vi "InitializeFunnelsByIndex.vi"(8 "error in (no error)":errorcluster, 10 "Funnels":string[](array[string]), 11 "Setting Database in":refnum<class "Setting Database.lvclass">) -> (0 "error out":errorcluster, 3 "Setting Database out":refnum<class "Setting Database.lvclass">)   [LabVIEW 2019, in "Setting Database.lvclass"]
uses:
  Setting Database.lvclass
  Funnel Settings/Funnel Settings.lvclass
  C:/Users/Albro/Documents/GitHub/AFM-Lithography/lvsrc/Classes/Settings/ObjectSettings/ObjectSettings.lvclass
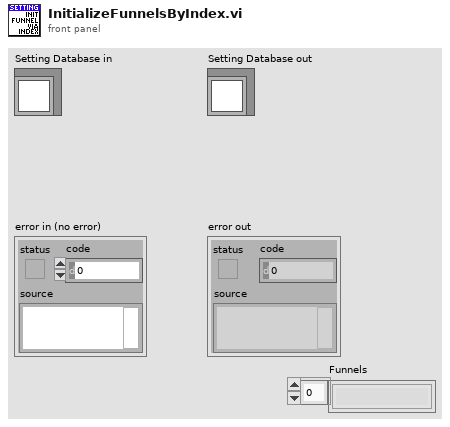
[diagram p1: front panel]
types:
  T1 = cluster{"Path":string, "Funnel":string, "Rectangle":string, "Dot":string}
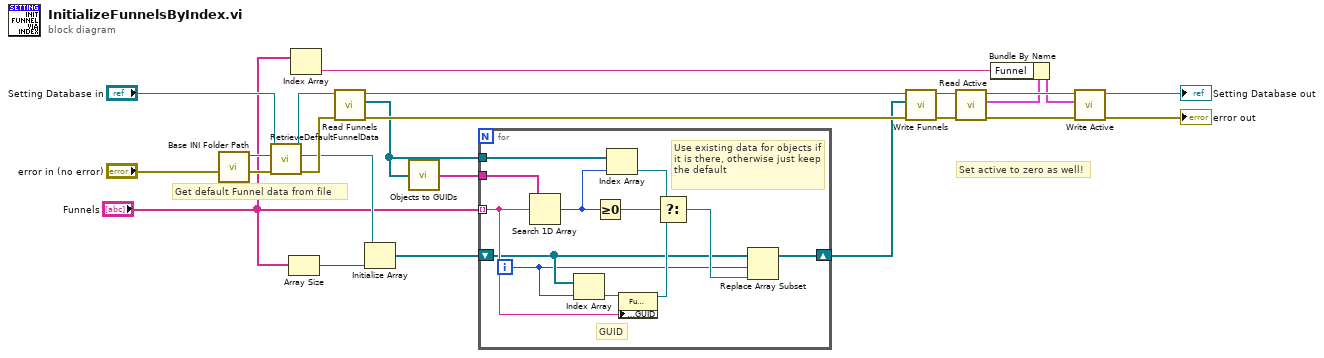
[diagram p0: block diagram]
diagram:
  # "Get default Funnel data from file"
  # "Set active to zero as well!"
  n1 = call "Base INI Folder Path.vi"() -> ("Base Path"=w8:path)  [unwired: 11 in]
  n2 = call "RetrieveDefaultFunnelData.vi"("error in (no error)"="error in (no error)", "Path"=w8, "Setting Database In"="Setting Database in") -> ("error out"=w16:errorcluster, "Funnel Settings.lvclass"=w11:refnum<class "Funnel Settings.lvclass">, "Setting Database Out"=w9:refnum<class "Setting Database.lvclass">)  [unwired: 6 in]
  n3 = Array Size(array="Funnels") -> (size(s)=w7:i32)
  n4 = Index Array(array="Funnels") -> (element=w1:string)  [unwired: 1 in]
  n5 = call "Read Funnels.vi"("error in (no error)"=w16, "Setting Database in"=w9) -> ("error out"=w13:errorcluster, "Funnels"=w6:refnum<class "Funnel Settings.lvclass">[], "Setting Database out"=w15:refnum<class "Setting Database.lvclass">)  [unwired: 7 in]
  n6 = Initialize Array(w11, w7) -> (w4:refnum<class "Funnel Settings.lvclass">[])
  n7 = call "Objects to GUIDs.vi"("Objects"=w6) -> ("GUIDs"=w5:string[])  [unwired: 3 in, 1 out]
  n8 = for {
    tunnel: w6 -> [w33]
    shift-right: [w35] -> w3
    shift-left: w4 -> [w25]
    tunnel: w5 -> [w32]
    tunnel: "Funnels" -> [w30] mode=indexing
    i -> [w24]
    # "GUID"
    # "Use existing data for objects if it is there, otherwise just keep the default"
    n9 = Search 1D Array(1D array=w32, element=w30) -> (index of element=w34:i32)  [unwired: 1 in]
    n10 = Index Array(array=w25, index=w24) -> (element=w31:refnum<class "Funnel Settings.lvclass">)
    n11 = Greater Or Equal To 0?(x=w34) -> (x >= 0?=w29:bool)
    n12 = Index Array(array=w33, index=w34) -> (element=w28:refnum<class "Funnel Settings.lvclass">)
    n13 = property class="Funnel Settings.lvclass"(reference=w31, "Accessors:GUID"=w30) -> (reference out=w26:refnum<class "Funnel Settings.lvclass">)  [unwired: 1 in, 1 out]
    n14 = Select(t=w28, s=w29, f=w26) -> (s? t:f=w27:refnum<class "Funnel Settings.lvclass">)
    n15 = Replace Array Subset(array=w25, new element=w27, index=w24) -> (w35:refnum<class "Funnel Settings.lvclass">[])
  }
  n16 = call "Write Funnels.vi"("error in (no error)"=w13, "Funnels"=w3, "Setting Database in"=w15) -> ("error out"=w12:errorcluster, "Setting Database out"=w14:refnum<class "Setting Database.lvclass">)  [unwired: 7 in]
  n17 = call "Read Active.vi"("error in (no error)"=w12, "Setting Database in"=w14) -> ("error out"=w22:errorcluster, "Active"=w21:T1, "Setting Database out"=w23:refnum<class "Setting Database.lvclass">)  [unwired: 7 in]
  n18 = Bundle By Name(cluster=w21, "Funnel"=w1) -> (w20:T1)
  n19 = call "Write Active.vi"("error in (no error)"=w22, "Active"=w20, "Setting Database in"=w23) -> ("error out"=→"error out":errorcluster, "Setting Database out"=→"Setting Database out":refnum<class "Setting Database.lvclass">)  [unwired: 7 in]
